vi "null.vi"(1 "Exit Loop ID":i32=-1, 2 "This Loop ID":i32) -> ()   [LabVIEW 2011]
doc: "Null state VI - does nothing for one iteration (it'll set its own exit value to TRUE) and can optionally end a parallel loops's substate."
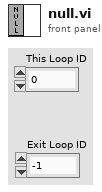
[diagram p1: front panel]
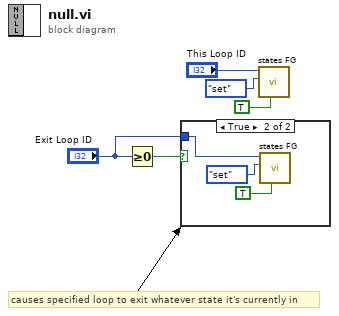
[diagram p0: block diagram]
diagram:
  # "causes specified loop to exit whatever state it's currently in"
  n1 = Greater Or Equal To 0?(x="Exit Loop ID") -> (x >= 0?=w1:bool)
  n2 = case shown="True" w1 {
    tunnel: "Exit Loop ID" -> [_ w6]
    frame False {
    }
    frame True {
      n3 = call "states FG.vi"("exit in"=TRUE, "menu (get)"=enum16{"set", "get"}."set", "Loop ID"=w6) -> ()  [unwired: 5 in, 4 out]
    }
  }
  n4 = call "states FG.vi"("exit in"=TRUE, "menu (get)"=enum16{"set", "get"}."set", "Loop ID"="This Loop ID") -> ()  [unwired: 5 in, 4 out]
